vi "Medulla_ATE_SoftFP.vi"(0 "reference in":refnum<class "Medulla_ATE.lvclass">, 2 "Floating":bool, 5 "error in (no error)":errorcluster) -> (14 "reference out":refnum<class "Medulla_ATE.lvclass">, 19 "error out":errorcluster)   [LabVIEW 2022 SP3, in "Medulla_ATE.lvlib" / "Medulla_ATE.lvclass"]
uses:
  Medulla_ATE.lvclass
  Components/DUT_Handler_Base.lvlibp/DUT_Handler_Base.lvclass
  Components/Test_Base.lvlibp/Test_Base.lvclass
  Components/ViPER.lvlibp/ViPER.lvclass
  C:/Projects/Medulla/ViPER/Examples/Flux_Capacitor_Tester/Components/ViPER.lvlibp/ViPER.lvclass
panel:
  in  "Exit":bool caption="Blank"
  in  "Login":bool caption="Blank"
  in  "Abort":bool caption="Stop"
  in  "Start":bool
  in  "Spec":bool caption="Open"
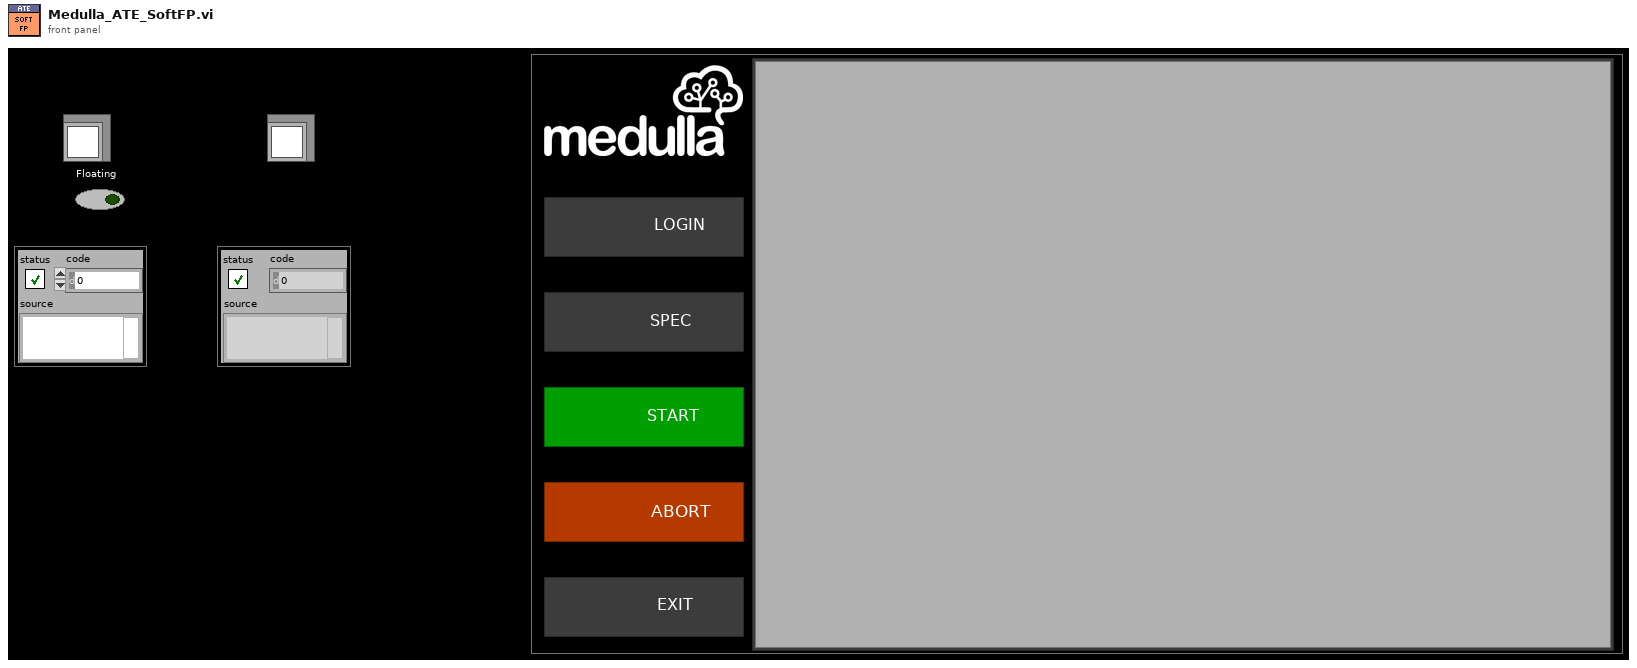
[diagram p1: front panel]
types:
  T1 = enum32{"Invalid", "Standard", "Closed", "Hidden", "Minimized", "Maximized"}
  T2 = typedef "Medulla_ATE.lvlib/Medulla_ATE.lvclass/ObjectAttributes.ctl" = cluster{"Config":T3, "DUT_Handler":refnum<class "DUT_Handler_Base.lvclass">, "MES":refnum<class "MES_Base.lvclass">, "TestView":refnum<class "TestView_Base.lvclass">, "TestClass":refnum<class "Test_Base.lvclass">}
  T3 = typedef "Medulla_ATE.lvlib/Medulla_ATE.lvclass/Config.ctl" = cluster{"ForceStart":bool, "ForceAbort":bool}
  T4 = enum8{"Enabled", "Disabled", "Disabled and Grayed Out"}
  T5 = enum16{"Load", "Cancel", "MoveIn", "MoveOut", "Abort", "Msg", "Enabled", "Disabled", "Fault", "Shutdown"}
  T6 = enum16{"Testing", "Pass", "Fail", "Abort", "Fault"}
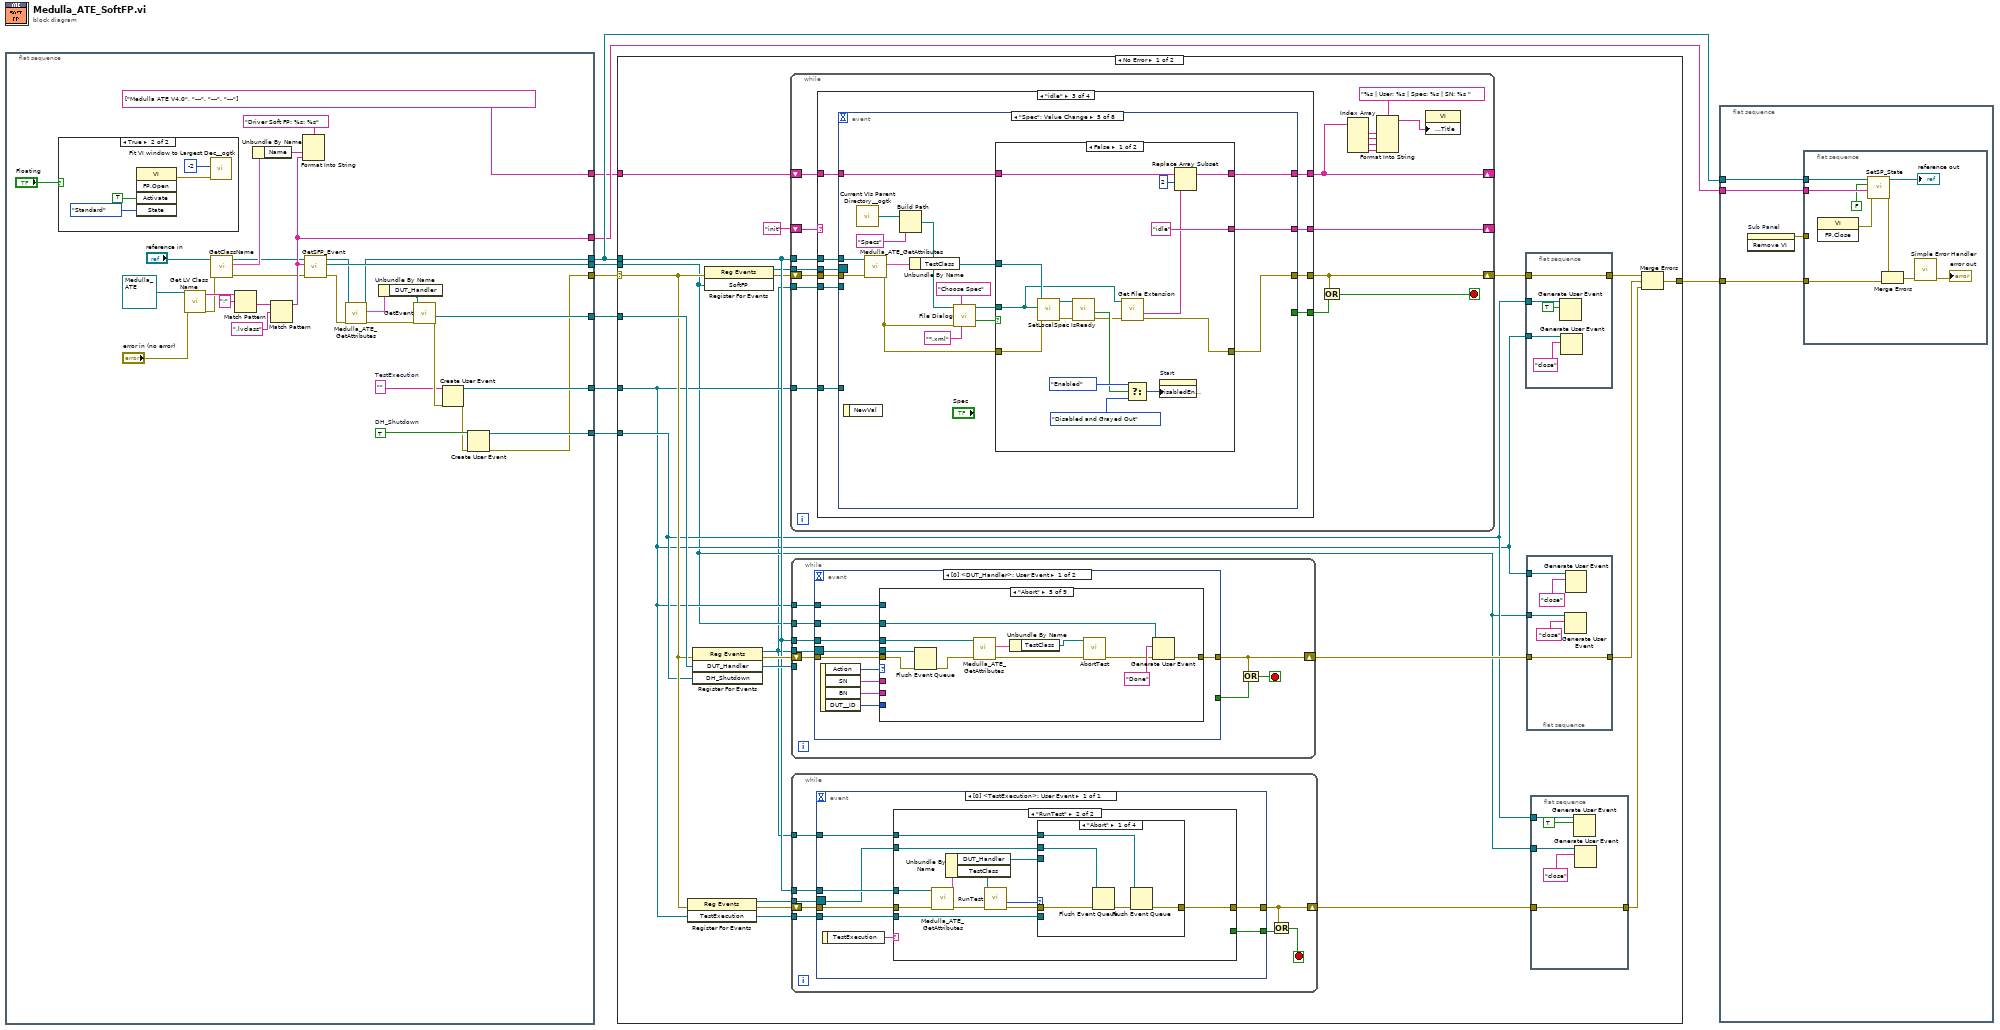
[diagram p0: block diagram]
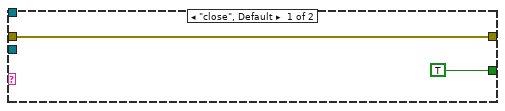
[diagram p3: hidden frame]
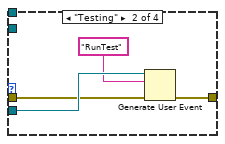
[diagram p4: hidden frame]
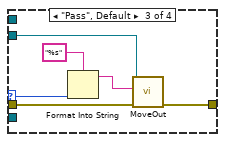
[diagram p5: hidden frame]
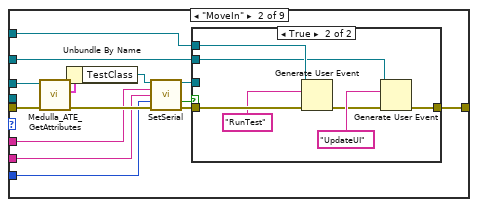
[diagram p8: hidden frame]
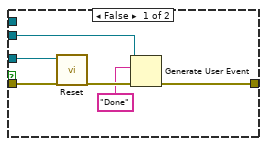
[diagram p9: hidden frame]
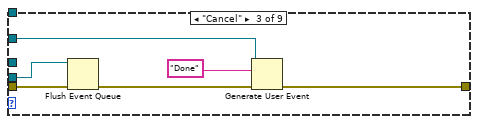
[diagram p10: hidden frame]
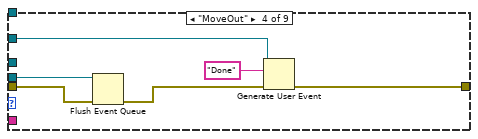
[diagram p11: hidden frame]
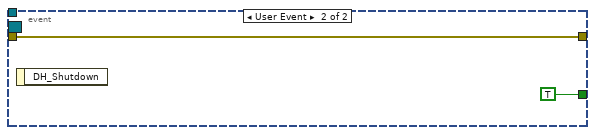
[diagram p16: hidden frame]
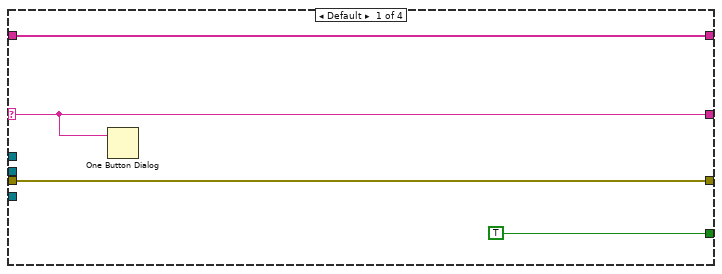
[diagram p17: hidden frame]
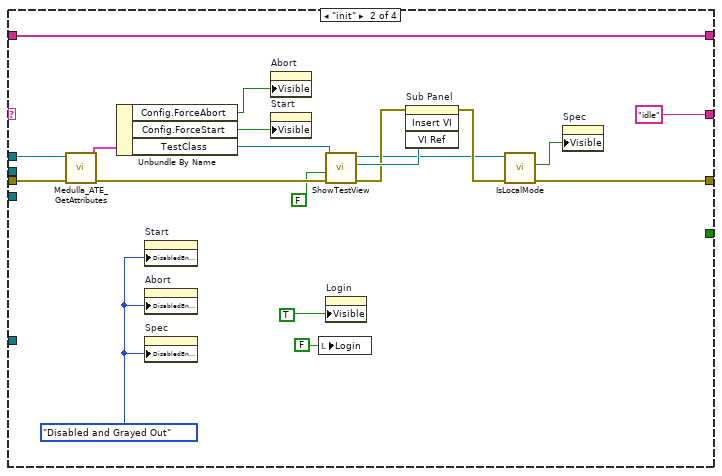
[diagram p18: hidden frame]
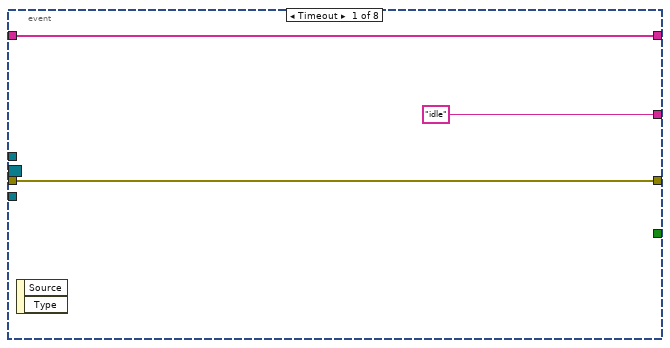
[diagram p19: hidden frame]
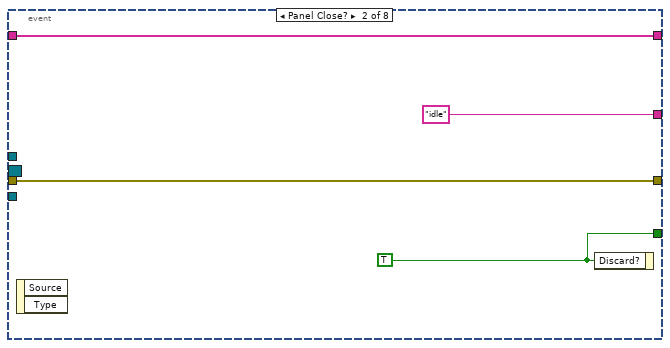
[diagram p20: hidden frame]
diagram:
  n1 = flat-sequence {
    tunnel: [w11] -> w9
    tunnel: [w23] -> w6
    tunnel: [w40] -> w7
    tunnel: [w31] -> w5
    tunnel: [w19] -> w4
    tunnel: [w15] -> w3
    tunnel: [w12] -> w2
    tunnel: [string[] ["Medulla ATE V4.0", "---", "---", "---"]] -> w1
    frame #0 {
      w14 = TRUE  # DH_Shutdown
      w16 = ""  # TestExecution
      n2 = case shown="True" "Floating" {
        frame False {
        }
        frame True {
          n3 = invoke class="VI" method="FP.Open"("Activate"=TRUE ("Activate?"), "State"=T1."Standard") -> (error out=w41:errorcluster)  [unwired: 3 in, 4 out]
          n4 = call <userlib>:"Fit VI window to Largest Dec__ogtk.vi"("error in (no error)"=w41, "border spacing (2 px)"=-2) -> ()  [unwired: 4 in, 2 out]
        }
      }
      n5 = call <vilib>:"Get LV Class Name.vi"("error in (no error)"="error in (no error)", "object"=refnum<class "Medulla_ATE.lvclass"> refnum ("reference")) -> ("error out"=w30:errorcluster, "class name"=w36:string)  [unwired: 8 in]
      n6 = call "GetClassName.vi"("error in (no error)"=w30, "reference in"="reference in") -> ("error out"=w29:errorcluster, "Details"=w28:cluster{"Name":string, "Class":string}, "reference out"=w26:refnum<class "Medulla_ATE.lvclass">)  [unwired: 7 in]
      n7 = Match Pattern(string=w36, regular expression=":") -> (after substring=w34:string)  [unwired: 1 in, 3 out]
      n8 = Unbundle By Name(w28) -> ("Name"=w38:string)
      n9 = Match Pattern(string=w34, regular expression=".lvclass") -> (before substring=w31:string)  [unwired: 1 in, 3 out]
      n10 = Format Into String(format string="Driver Soft FP: %s: %s", w38, w31) -> ()  [unwired: 2 in, 2 out]
      n11 = call-dynamic "GetSFP_Event.vi"("error in (no error)"=w29, "Ancestor"=w31, "reference in"=w26) -> ("error out"=w25:errorcluster, "SoftFP"=w40:refnum<user-event>, "reference out"=w24:refnum<class "Medulla_ATE.lvclass">)  [unwired: 6 in]
      n12 = call "Medulla_ATE_GetAttributes.vi"("error in (no error)"=w25, "reference in"=w24) -> ("error out"=w22:errorcluster, "Data"=w21:T2, "reference out"=w23:refnum<class "Medulla_ATE.lvclass">)  [unwired: 6 in, 1 out]
      n13 = Unbundle By Name(w21) -> ("DUT_Handler"=w20:refnum<class "DUT_Handler_Base.lvclass">)
      n14 = call-dynamic "GetEvent.vi"("error in (no error)"=w22, "reference in"=w20) -> ("error out"=w17:errorcluster, "DUT_Handler"=w19:refnum<user-event>)  [unwired: 6 in, 1 out]
      n15 = Create User Event(user event datatype=w16, error in=w17) -> (user event=w15:refnum<user-event>, error out=w13:errorcluster)
      n16 = Create User Event(user event datatype=w14, error in=w13) -> (user event=w12:refnum<user-event>, error out=w11:errorcluster)
    }
  }
  n17 = case shown="No Error" w9 {
    selector: w9 -> [w57 w406]
    tunnel: [w52 w406] -> w8
    tunnel: w6 -> [w60 _]
    tunnel: w7 -> [w47 _]
    tunnel: w4 -> [w63 _]
    tunnel: w3 -> [w53 _]
    tunnel: w2 -> [w55 _]
    tunnel: w1 -> [w46 _]
    frame No Error {
      n18 = register-events(error in=w57, w53) -> (reference out=w62:refnum<event-registration>, error out=w61:errorcluster)  [unwired: 1 in]
      n19 = register-events(error in=w57, w63, w55) -> (reference out=w45:refnum<event-registration>, error out=w64:errorcluster)  [unwired: 1 in]
      n20 = register-events(error in=w57, w47) -> (reference out=w48:refnum<event-registration>, error out=w56:errorcluster)  [unwired: 1 in]
      n21 = while {
        shift-right: [w217] -> w59
        shift-left: w56 -> [w219]
        tunnel: w60 -> [w218]
        shift-right: [w213] -> _
        shift-left: "init" -> [w214]
        tunnel: w53 -> [w212]
        tunnel: w48 -> [w211]
        shift-right: [w203] -> _
        shift-left: w46 -> [w210]
        tunnel: w45 -> [w202]
        stop <- w216 stop-if-true
        n22 = case shown="\"idle\"" w214 {
          selector: w214 -> [w221 _ _ _]
          tunnel: w219 -> [w222 w241 w252 w402]
          tunnel: w218 -> [_ w240 w251 w401]
          tunnel: [w222 w238 w250 w400] -> w217
          tunnel: [TRUE ("Discard?") _ w249 _] -> w215
          tunnel: [w221 "idle" w248 "idle"] -> w213
          tunnel: w212 -> [_ _ w247 _]
          tunnel: w211 -> [_ _ w246 _]
          tunnel: w210 -> [w220 w224 w245 w398]
          tunnel: [w220 w224 w244 w398] -> w203
          tunnel: w202 -> [_ _ w243 _]
          frame Default {
            n23 = One Button Dialog(message=w221) -> ()  [unwired: 1 in, 1 out]
          }
          frame "init" {
            w226 = T4."Disabled and Grayed Out" ("Disabled")
            n24 = call "Medulla_ATE_GetAttributes.vi"("error in (no error)"=w241, "reference in"=w240) -> ("error out"=w237:errorcluster, "Data"=w239:T2)  [unwired: 6 in, 2 out]
            n25 = Unbundle By Name(w239) -> ("Config.ForceAbort"=w230:bool, "Config.ForceStart"=w229:bool, "TestClass"=w236:refnum<class "Test_Base.lvclass">)
            n26 = property on="Start" class="Bool"("DisabledEnum"=w226) -> ()  [unwired: 2 in, 2 out]
            n27 = property on="Abort" class="Bool"("DisabledEnum"=w226) -> ()  [unwired: 2 in, 2 out]
            n28 = property on="Spec" class="Bool"("DisabledEnum"=w226) -> ()  [unwired: 2 in, 2 out]
            n29 = property on="Abort" class="Bool"("Visible"=w230) -> ()  [unwired: 2 in, 2 out]
            n30 = property on="Start" class="Bool"("Visible"=w229) -> ()  [unwired: 2 in, 2 out]
            n31 = local write "Login"(FALSE ("Login")) -> ()
            n32 = call-dynamic "ShowTestView.vi"("error in (no error)"=w237, "Floating"=FALSE, "reference in"=w236) -> ("error out"=w233:errorcluster, "UI"=w234:refnum<vi>, "reference in"=w231:refnum<class "Test_Base.lvclass">)  [unwired: 6 in]
            n33 = property on="Login" class="Bool (strict)"("Visible"=TRUE) -> ()  [unwired: 2 in, 2 out]
            n34 = invoke on="Sub Panel" class="SubPnl" method="Insert VI"(error in=w233, "VI Ref"=w234) -> (error out=w232:errorcluster)  [unwired: 2 in, 3 out]
            n35 = call-dynamic "IsLocalMode.vi"("error in (no error)"=w232, "reference in"=w231) -> ("error out"=w238:errorcluster, "Is Local"=w228:bool)  [unwired: 7 in, 1 out]
            n36 = property on="Spec" class="Bool"("Visible"=w228) -> ()  [unwired: 2 in, 2 out]
          }
          frame "idle" {
            n37 = event shown="[4] \"Spec\": Value Change" {
              selector: w246 -> [_ _ _ _ _ _ _ _]
              dyn-events: _ -> [_ _ _ _ _ _ _ _]
              timeout: _ -> [_ _ _ _ _ _ _ _]
              tunnel: w252 -> [w255 w259 w268 w302 w353 w381 w392 w395]
              tunnel: [w255 w259 w266 w299 w349 w376 w388 w395] -> w250
              tunnel: [_ w258 w265 _ _ _ _ TRUE ("Discard?")] -> w249
              tunnel: w251 -> [_ _ w264 w301 w352 w380 w391 _]
              tunnel: ["idle" "idle" w262 "idle" w344 "idle" "idle" "exit"] -> w248
              tunnel: w247 -> [_ _ w263 _ _ _ _ _]
              tunnel: [w253 w256 w260 w295 w338 w373 w387 w394] -> w244
              tunnel: w245 -> [w253 w256 w261 w296 w339 w373 w387 w394]
              tunnel: w243 -> [_ _ _ _ _ _ w384 _]
              event Timeout {
                n38 = event-data() -> ()  [unwired: 1 in, 2 out]
              }
              event Panel Close? {
                w258 = TRUE ("Discard?")
                n39 = event-data() -> ()  [unwired: 1 in, 2 out]
                n40 = event-data("Discard?"=w258) -> ()  [unwired: 1 in, 1 out]
              }
              event User Event {
                n41 = event-data() -> ("SoftFP"=w267:string)  [unwired: 1 in]
                n42 = case shown="\"Done\"" w267 {
                  tunnel: w268 -> [w273 w286 w292]
                  tunnel: [w273 w287 w292] -> w266
                  tunnel: [_ _ TRUE ("Discard?")] -> w265
                  tunnel: w264 -> [_ w284 _]
                  tunnel: w263 -> [_ _ _]
                  tunnel: ["idle" "idle" "exit"] -> w262
                  tunnel: w261 -> [w269 w281 w289]
                  tunnel: [w269 w274 w289] -> w260
                  frame "Done" {
                    w270 = T4."Enabled" ("Disabled")
                    n43 = property on="Spec" class="Bool"("DisabledEnum"=w270) -> ()  [unwired: 2 in, 2 out]
                    n44 = property on="Start" class="Bool"("DisabledEnum"=w270) -> ()  [unwired: 2 in, 2 out]
                    n45 = property on="Abort" class="Bool"("DisabledEnum"=T4."Disabled and Grayed Out" ("Disabled")) -> ()  [unwired: 2 in, 2 out]
                    n46 = property on="Login" class="Bool (strict)"("DisabledEnum"=w270) -> ()  [unwired: 2 in, 2 out]
                  }
                  frame "UpdateUI" {
                    n47 = call "Medulla_ATE_GetAttributes.vi"("error in (no error)"=w286, "reference in"=w284) -> ("error out"=w285:errorcluster, "Data"=w283:T2)  [unwired: 6 in, 2 out]
                    n48 = Unbundle By Name(w283) -> ("TestClass"=w282:refnum<class "Test_Base.lvclass">)
                    n49 = call-dynamic "GetUUTIndex.vi"("error in (no error)"=w285, "reference in"=w282) -> ("error out"=w287:errorcluster, "Serial"=w279:string, "Index"=w276:i32)  [unwired: 5 in, 2 out]
                    n50 = Number To Decimal String(number=w276) -> (decimal integer string=w275:string)  [unwired: 1 in]
                    n51 = Replace Array Subset(array=w281, new element=w279, index=3) -> (w278:string[])
                    n52 = Replace Array Subset(array=w278, new element=w275, index=4) -> (w274:string[])
                  }
                  frame "close", Default {
                  }
                }
              }
              event "Login": Value Change {
                n53 = event-data() -> ()  [unwired: 1 in, 1 out]
                n54 = case shown="True" "Login" {
                  tunnel: w302 -> [w308 w322]
                  tunnel: w301 -> [w307 w321]
                  tunnel: [w306 w316] -> w298
                  tunnel: [w304 w312] -> w297
                  frame False {
                    w305 = T4."Disabled and Grayed Out" ("Disabled")
                    n55 = call "Medulla_ATE_GetAttributes.vi"("error in (no error)"=w308, "reference in"=w307) -> ("error out"=w311:errorcluster, "Data"=w310:T2)  [unwired: 6 in, 2 out]
                    n56 = Unbundle By Name(w310) -> ("TestClass"=w309:refnum<class "Test_Base.lvclass">)
                    n57 = call-dynamic "Logout.vi"("error in (no error)"=w311, "reference in"=w309) -> ("error out"=w306:errorcluster, "reference in"=w304:refnum<class "Test_Base.lvclass">)  [unwired: 8 in]
                    n58 = property on="Abort" class="Bool"("DisabledEnum"=w305) -> ()  [unwired: 2 in, 2 out]
                    n59 = property on="Spec" class="Bool"("DisabledEnum"=w305) -> ()  [unwired: 2 in, 2 out]
                    n60 = property on="Start" class="Bool"("DisabledEnum"=w305) -> ()  [unwired: 2 in, 2 out]
                  }
                  frame True {
                    n61 = call "Medulla_ATE_GetAttributes.vi"("error in (no error)"=w322, "reference in"=w321) -> ("error out"=w318:errorcluster, "Data"=w317:T2)  [unwired: 6 in, 2 out]
                    n62 = Unbundle By Name(w317) -> ("TestClass"=w319:refnum<class "Test_Base.lvclass">)
                    n63 = call-dynamic "Login.vi"("error in (no error)"=w318, "reference in"=w319) -> ("error out"=w320:errorcluster, "cancelled"=w313:bool, "valid"=w314:bool, "reference in"=w315:refnum<class "Test_Base.lvclass">)  [unwired: 6 in]
                    n64 = case shown="False" w314 {
                      tunnel: w320 -> [w326 w337]
                      tunnel: [w326 w336] -> w316
                      tunnel: w315 -> [w323 w335]
                      tunnel: w313 -> [w327 _]
                      tunnel: [w323 w329] -> w312
                      frame False {
                        w325 = T4."Disabled and Grayed Out" ("Disabled")
                        n65 = case shown="False" w327 {
                          frame False {
                            n66 = One Button Dialog(message="Invalid User") -> ()  [unwired: 1 in, 1 out]
                          }
                          frame True {
                          }
                        }
                        n67 = local write "Login"(FALSE ("Login")) -> ()
                        n68 = property on="Start" class="Bool"("DisabledEnum"=w325) -> ()  [unwired: 2 in, 2 out]
                        n69 = property on="Abort" class="Bool"("DisabledEnum"=w325) -> ()  [unwired: 2 in, 2 out]
                        n70 = property on="Spec" class="Bool"("DisabledEnum"=w325) -> ()  [unwired: 2 in, 2 out]
                      }
                      frame True {
                        w330 = T4."Disabled and Grayed Out" ("Disabled")
                        n71 = call-dynamic "IsReady.vi"("error in (no error)"=w337, "reference in"=w335) -> ("error out"=w336:errorcluster, "OK"=w334:bool, "reference in"=w329:refnum<class "Test_Base.lvclass">)  [unwired: 7 in]
                        n72 = property on="Spec" class="Bool"("DisabledEnum"=T4."Enabled" ("Disabled")) -> ()  [unwired: 2 in, 2 out]
                        n73 = Select(t=T4."Enabled" ("Disabled"), s=w334, f=w330) -> (s? t:f=w332:T4)
                        n74 = property on="Start" class="Bool"("DisabledEnum"=w332) -> ()  [unwired: 2 in, 2 out]
                        n75 = property on="Abort" class="Bool"("DisabledEnum"=w330) -> ()  [unwired: 2 in, 2 out]
                      }
                    }
                  }
                }
                n76 = call-dynamic "GetUser.vi"("reference in"=w297, "error in (no error)"=w298) -> ("User"=w294:string, "error out"=w299:errorcluster)  [unwired: 15 in, 1 out]
                n77 = Replace Array Subset(array=w296, new element=w294, index=1 ("disabled index (col)")) -> (w295:string[])
              }
              event "Spec": Value Change {
                n78 = event-data() -> ()  [unwired: 1 in, 1 out]
                n79 = call <userlib>:"Current VIs Parent Directory__ogtk.vi"() -> ("Parent Directory (+ Relative)"=w348:path)  [unwired: 5 in]
                n80 = call "Medulla_ATE_GetAttributes.vi"("error in (no error)"=w353, "reference in"=w352) -> ("error out"=w341:errorcluster, "Data"=w351:T2)  [unwired: 6 in, 2 out]
                n81 = Build Path(base path=w348, name or relative path="Specs") -> (appended path=w340:path)
                n82 = Unbundle By Name(w351) -> ("TestClass"=w350:refnum<class "Test_Base.lvclass">)
                n83 = call "File Dialog"("start path"=w340, "prompt"="Choose Spec", "error in"=w341, "pattern (all files)"="*.xml") -> ("selected path"=w345:path, "cancelled"=w346:bool)  [unwired: 8 in, 2 out]
                n84 = case shown="False" w346 {
                  tunnel: w350 -> [w369 _]
                  tunnel: [w359 w372] -> w349
                  tunnel: w341 -> [w368 w372]
                  tunnel: w345 -> [w358 _]
                  tunnel: ["idle" "idle"] -> w344
                  tunnel: w339 -> [w357 w370]
                  tunnel: [w355 w370] -> w338
                  frame False {
                    n85 = call-dynamic "SetLocalSpec.vi"("error in (no error)"=w368, "Path"=w358, "reference in"=w369) -> ("error out"=w366:errorcluster, "reference in"=w365:refnum<class "Test_Base.lvclass">)  [unwired: 7 in]
                    n86 = call-dynamic "IsReady.vi"("error in (no error)"=w366, "reference in"=w365) -> ("error out"=w360:errorcluster, "OK"=w362:bool)  [unwired: 7 in, 1 out]
                    n87 = call <vilib>:"Get File Extension.vi"("error in (no error)"=w360, "file"=w358) -> ("error out"=w359:errorcluster, "filename without extension"=w354:string)  [unwired: 5 in, 3 out]
                    n88 = Select(t=T4."Enabled" ("Disabled"), s=w362, f=T4."Disabled and Grayed Out" ("Disabled")) -> (s? t:f=w361:T4)
                    n89 = property on="Start" class="Bool"("DisabledEnum"=w361) -> ()  [unwired: 2 in, 2 out]
                    n90 = Replace Array Subset(array=w357, new element=w354, index=2 ("index (row)")) -> (w355:string[])
                  }
                  frame True {
                  }
                }
              }
              event "Start": Value Change {
                n91 = event-data() -> ()  [unwired: 1 in, 6 out]
                n92 = call "Medulla_ATE_GetAttributes.vi"("error in (no error)"=w381, "reference in"=w380) -> ("error out"=w377:errorcluster, "Data"=w379:T2)  [unwired: 6 in, 2 out]
                n93 = Unbundle By Name(w379) -> ("DUT_Handler"=w375:refnum<class "DUT_Handler_Base.lvclass">)
                n94 = call-dynamic "MoveIn.vi"("error in (no error)"=w377, "reference in"=w375) -> ("error out"=w376:errorcluster, "OK"=w374:bool)  [unwired: 7 in, 1 out]
                n95 = case shown="True" w374 {
                  frame False {
                  }
                  frame True {
                    w382 = T4."Disabled and Grayed Out" ("Disabled")
                    n96 = property on="Start" class="Bool"("DisabledEnum"=w382) -> ()  [unwired: 2 in, 2 out]
                    n97 = property on="Spec" class="Bool"("DisabledEnum"=w382) -> ()  [unwired: 2 in, 2 out]
                    n98 = property on="Abort" class="Bool"("DisabledEnum"=T4."Enabled" ("Disabled")) -> ()  [unwired: 2 in, 2 out]
                    n99 = property on="Login" class="Bool (strict)"("DisabledEnum"=w382) -> ()  [unwired: 2 in, 2 out]
                  }
                }
              }
              event "Abort": Value Change {
                n100 = event-data() -> ()  [unwired: 1 in, 6 out]
                n101 = call "Medulla_ATE_GetAttributes.vi"("error in (no error)"=w392, "reference in"=w391) -> ("error out"=w386:errorcluster, "Data"=w390:T2)  [unwired: 6 in, 2 out]
                n102 = Unbundle By Name(w390) -> ("DUT_Handler"=w389:refnum<class "DUT_Handler_Base.lvclass">)
                n103 = Flush Event Queue(0:w384, 3:w386) -> (11:w385:errorcluster)  [unwired: 4 in, 2 out]
                n104 = call-dynamic "Abort.vi"("reference in"=w389, "error in (no error)"=w385) -> ("error out"=w388:errorcluster)  [unwired: 16 in, 1 out]
              }
              event "Exit": Value Change {
                n105 = event-data() -> ()  [unwired: 1 in, 6 out]
              }
            }
          }
          frame "exit" {
            n106 = call "Medulla_ATE_GetAttributes.vi"("error in (no error)"=w402, "reference in"=w401) -> ("error out"=w404:errorcluster, "Data"=w405:T2)  [unwired: 6 in, 2 out]
            n107 = Unbundle By Name(w405) -> ("TestClass"=w403:refnum<class "Test_Base.lvclass">)
            n108 = call-dynamic "Shutdown.vi"("error in (no error)"=w404, "reference in"=w403) -> ("error out"=w400:errorcluster)  [unwired: 8 in, 1 out]
          }
        }
        n109 = Or(x=w217, y=w215) -> (x .or. y?=w216:bool)
        n110 = Index Array(array=w203) -> (element #1=w209:string, element #2=w208:string, element #3=w207:string, element #4=w206:string)  [unwired: 4 in]
        n111 = Format Into String(format string="%s | User: %s | Spec: %s | SN: %s ", w209, w208, w207, w206) -> (resulting string=w204:string)  [unwired: 2 in, 1 out]
        n112 = property class="VI"("Front Panel.Title"=w204) -> ()  [unwired: 2 in, 2 out]
      }
      n113 = while {
        shift-right: [w130] -> w58
        shift-left: w64 -> [w134]
        tunnel: w63 -> [_]
        tunnel: w45 -> [w133]
        tunnel: w60 -> [w132]
        tunnel: w47 -> [w131]
        tunnel: w53 -> [w127]
        stop <- w129 stop-if-true
        n114 = event shown="[0] <DUT_Handler>: User Event" {
          selector: w133 -> [w135 _]
          dyn-events: _ -> [_ _]
          timeout: _ -> [_ _]
          tunnel: w134 -> [w139 w201]
          tunnel: w132 -> [w140 _]
          tunnel: [w138 w201] -> w130
          tunnel: w131 -> [w137 _]
          tunnel: [_ TRUE] -> w128
          tunnel: w127 -> [w136 _]
          event User Event {
            n115 = event-data() -> ("Action"=w144:T5, "SN"=w143:string, "BN"=w142:string, "DUT__ID"=w141:u32)  [unwired: 1 in]
            n116 = case shown="\"Abort\"" w144 {
              tunnel: w143 -> [_ w152 _ _ _ _ _ _ _]
              tunnel: w142 -> [_ w153 _ _ _ _ _ _ _]
              tunnel: w141 -> [_ w154 _ _ _ _ _ _ _]
              tunnel: w139 -> [w145 w158 w175 w181 w187 w196 w197 w198 w199]
              tunnel: w140 -> [_ w156 _ _ w192 _ _ _ _]
              tunnel: [w145 w147 w178 w184 w190 w196 w197 w198 w199] -> w138
              tunnel: w137 -> [_ w148 w176 w182 w189 _ _ _ _]
              tunnel: w136 -> [_ w146 _ _ _ _ _ _ _]
              tunnel: w135 -> [_ _ w173 w179 w185 _ _ _ _]
              frame "Load", Default {
              }
              frame "MoveIn" {
                n117 = call "Medulla_ATE_GetAttributes.vi"("error in (no error)"=w158, "reference in"=w156) -> ("error out"=w157:errorcluster, "Data"=w159:T2)  [unwired: 6 in, 2 out]
                n118 = Unbundle By Name(w159) -> ("TestClass"=w155:refnum<class "Test_Base.lvclass">)
                n119 = call-dynamic "SetSerial.vi"("reference in"=w155, "SN"=w152, "BN"=w153, "UUT_Index"=w154, "error in (no error)"=w157) -> ("reference in"=w149:refnum<class "Test_Base.lvclass">, "OK"=w151:bool, "error out"=w150:errorcluster)  [unwired: 8 in]
                n120 = case shown="True" w151 {
                  tunnel: w150 -> [w165 w172]
                  tunnel: w149 -> [w164 _]
                  tunnel: [w162 w167] -> w147
                  tunnel: w148 -> [w160 w166]
                  tunnel: w146 -> [_ w171]
                  frame False {
                    n121 = call-dynamic "Reset.vi"("reference in"=w164, "error in (no error)"=w165) -> ("error out"=w163:errorcluster)  [unwired: 16 in, 1 out]
                    n122 = Generate User Event(user event=w160, event data cluster="Done" ("event data"), error in=w163) -> (error out=w162:errorcluster)  [unwired: 1 in, 1 out]
                  }
                  frame True {
                    n123 = Generate User Event(user event=w171, event data cluster="RunTest" ("event data"), error in=w172) -> (error out=w168:errorcluster)  [unwired: 1 in, 1 out]
                    n124 = Generate User Event(user event=w166, event data cluster="UpdateUI" ("event data"), error in=w168) -> (error out=w167:errorcluster)  [unwired: 1 in, 1 out]
                  }
                }
              }
              frame "Cancel" {
                n125 = Flush Event Queue(0:w173, 3:w175) -> (11:w174:errorcluster)  [unwired: 4 in, 2 out]
                n126 = Generate User Event(user event=w176, event data cluster="Done" ("event data"), error in=w174) -> (error out=w178:errorcluster)  [unwired: 1 in, 1 out]
              }
              frame "MoveOut" {
                n127 = Flush Event Queue(0:w179, 3:w181) -> (11:w180:errorcluster)  [unwired: 4 in, 2 out]
                n128 = Generate User Event(user event=w182, event data cluster="Done" ("event data"), error in=w180) -> (error out=w184:errorcluster)  [unwired: 1 in, 1 out]
              }
              frame "Abort" {
                n129 = Flush Event Queue(0:w185, 3:w187) -> (11:w186:errorcluster)  [unwired: 4 in, 2 out]
                n130 = call "Medulla_ATE_GetAttributes.vi"("error in (no error)"=w186, "reference in"=w192) -> ("error out"=w195:errorcluster, "Data"=w194:T2)  [unwired: 6 in, 2 out]
                n131 = Unbundle By Name(w194) -> ("TestClass"=w193:refnum<class "Test_Base.lvclass">)
                n132 = call-dynamic "AbortTest.vi"("error in (no error)"=w195, "reference in"=w193) -> ("error out"=w188:errorcluster)  [unwired: 8 in, 1 out]
                n133 = Generate User Event(user event=w189, event data cluster="Done" ("event data"), error in=w188) -> (error out=w190:errorcluster)  [unwired: 1 in, 1 out]
              }
              frame "Msg" {
              }
              frame "Enabled" {
              }
              frame "Disabled" {
              }
              frame "Fault" {
              }
            }
          }
          event User Event {
            n134 = event-data() -> ()  [unwired: 1 in, 1 out]
          }
        }
        n135 = Or(x=w130, y=w128) -> (x .or. y?=w129:bool)
      }
      n136 = while {
        tunnel: w62 -> [w88]
        tunnel: w53 -> [w87]
        shift-right: [w84] -> w54
        shift-left: w61 -> [w86]
        tunnel: w60 -> [w85]
        tunnel: w45 -> [w81]
        stop <- w82 stop-if-true
        n137 = event shown="[0] <TestExecution>: User Event" {
          selector: w88 -> [w90]
          dyn-events: _ -> [_]
          timeout: _ -> [_]
          tunnel: w87 -> [w93]
          tunnel: w86 -> [w96]
          tunnel: [w95] -> w84
          tunnel: w85 -> [w94]
          tunnel: [w91] -> w83
          tunnel: w81 -> [w89]
          event User Event {
            n138 = event-data() -> ("TestExecution"=w92:string)  [unwired: 1 in]
            n139 = case shown="\"RunTest\"" w92 {
              tunnel: w96 -> [w98 w104]
              tunnel: [w98 w103] -> w95
              tunnel: w94 -> [_ w102]
              tunnel: w93 -> [_ w101]
              tunnel: [TRUE _] -> w91
              tunnel: w90 -> [_ w100]
              tunnel: w89 -> [_ w99]
              frame "close", Default {
              }
              frame "RunTest" {
                n140 = call "Medulla_ATE_GetAttributes.vi"("error in (no error)"=w104, "reference in"=w102) -> ("error out"=w110:errorcluster, "Data"=w109:T2)  [unwired: 6 in, 2 out]
                n141 = Unbundle By Name(w109) -> ("DUT_Handler"=w105:refnum<class "DUT_Handler_Base.lvclass">, "TestClass"=w108:refnum<class "Test_Base.lvclass">)
                n142 = call-dynamic "RunTest.vi"("error in (no error)"=w110, "reference in"=w108) -> ("error out"=w107:errorcluster, "State"=w106:T6)  [unwired: 7 in, 1 out]
                n143 = case shown="\"Abort\"" w106 {
                  selector: w106 -> [_ _ w122 _]
                  tunnel: w107 -> [w115 w118 w125 w126]
                  tunnel: w105 -> [_ _ w123 _]
                  tunnel: [w112 w117 w124 w126] -> w103
                  tunnel: w101 -> [_ w119 _ _]
                  tunnel: w100 -> [w114 _ _ _]
                  tunnel: w99 -> [w111 _ _ _]
                  frame "Abort" {
                    n144 = Flush Event Queue(0:w114, 3:w115) -> (11:w113:errorcluster)  [unwired: 4 in, 2 out]
                    n145 = Flush Event Queue(0:w111, 3:w113) -> (11:w112:errorcluster)  [unwired: 4 in, 2 out]
                  }
                  frame "Testing" {
                    n146 = Generate User Event(user event=w119, event data cluster="RunTest", error in=w118) -> (error out=w117:errorcluster)  [unwired: 1 in, 1 out]
                  }
                  frame "Pass", Default {
                    n147 = Format Into String(format string="%s", w122) -> (resulting string=w120:string)  [unwired: 2 in, 1 out]
                    n148 = call-dynamic "MoveOut.vi"("error in (no error)"=w125, "Destination"=w120, "reference in"=w123) -> ("error out"=w124:errorcluster)  [unwired: 7 in, 1 out]
                  }
                  frame "Fault" {
                  }
                }
              }
            }
          }
        }
        n149 = Or(x=w84, y=w83) -> (x .or. y?=w82:bool)
      }
      n150 = flat-sequence {
        tunnel: w59 -> [w80]
        tunnel: [w80] -> w51
        tunnel: w55 -> [w79]
        tunnel: w53 -> [w77]
        frame #0 {
          n151 = Generate User Event(user event=w79, event data cluster=TRUE ("event data")) -> ()  [unwired: 2 in, 2 out]
          n152 = Generate User Event(user event=w77, event data cluster="close" ("event data")) -> ()  [unwired: 2 in, 2 out]
        }
      }
      n153 = flat-sequence {
        tunnel: [w75] -> w50
        tunnel: w58 -> [w75]
        tunnel: w53 -> [w74]
        tunnel: w47 -> [w73]
        frame #0 {
          n154 = Generate User Event(user event=w73, event data cluster="close" ("event data")) -> ()  [unwired: 2 in, 2 out]
          n155 = Generate User Event(user event=w74, event data cluster="close" ("event data")) -> ()  [unwired: 2 in, 2 out]
        }
      }
      n156 = flat-sequence {
        tunnel: [w70] -> w49
        tunnel: w54 -> [w70]
        tunnel: w55 -> [w68]
        tunnel: w47 -> [w67]
        frame #0 {
          n157 = Generate User Event(user event=w68, event data cluster=TRUE ("event data")) -> ()  [unwired: 2 in, 2 out]
          n158 = Generate User Event(user event=w67, event data cluster="close" ("event data")) -> ()  [unwired: 2 in, 2 out]
        }
      }
      n159 = Merge Errors(w51, w50, w49) -> (w52:errorcluster)
    }
    frame Error {
    }
  }
  n160 = flat-sequence {
    tunnel: w8 -> [w408]
    tunnel: w6 -> [w409]
    tunnel: w5 -> [w410]
    frame #0 {
      n161 = invoke on="Sub Panel" class="SubPnl" method="Remove VI"() -> (error out=w407:errorcluster)  [unwired: 3 in, 2 out]
      n162 = flat-sequence {
        tunnel: w410 -> [w415]
        tunnel: w409 -> [w413]
        tunnel: w408 -> [w411]
        tunnel: w407 -> [_]
        frame #0 {
          n163 = invoke class="VI" method="FP.Close"() -> (error out=w417:errorcluster)  [unwired: 3 in, 2 out]
          n164 = call "SetSP_State.vi"("error in (no error)"=w417, "Ancestor"=w415, "SP Open"=FALSE, "reference in"=w413) -> ("error out"=w416:errorcluster, "reference out"=→"reference out":refnum<class "Medulla_ATE.lvclass">)  [unwired: 6 in]
          n165 = Merge Errors(w416, w411) -> (w419:errorcluster)
          n166 = call <vilib>:"Simple Error Handler.vi"("error in (no error)"=w419) -> ("error out"=→"error out":errorcluster)  [unwired: 4 in, 4 out]
        }
      }
    }
  }
